vi "SI657_From_trubine.vi"(0 "From Turbine SI656":T1, 2 "From Turbine SI657":T2, 5 "error in (no error)":errorcluster, 8 "SI657.lvclass":refnum<class "SI657.lvclass">, 10 "SI656.lvclass":refnum<class "SI656.lvclass">) -> (9 "SI657.lvclass out":refnum<class "SI657.lvclass">, 11 "SI656 out":refnum<class "SI656.lvclass">, 14 "PG SP-Grad":dbl, 15 "PG SP lift-up":dbl, 16 "PG eff SP":dbl, 17 "Switch Ps-Ps_d":dbl, 18 "PG target SP":dbl, 19 "error out":errorcluster)   [LabVIEW 2022 SP3, in "SI657.lvclass"]
uses:
  SI657.lvclass
  SI657.lvclass/SI657.ctl
  SI656/SI656.lvclass
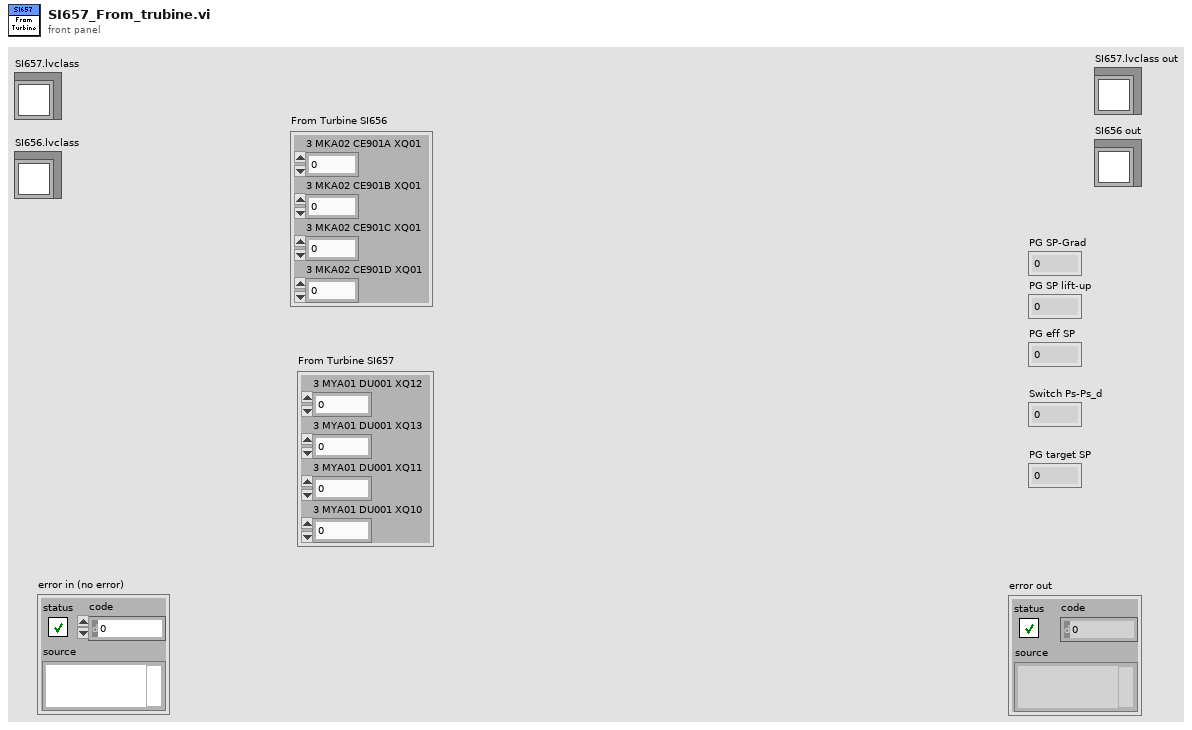
[diagram p1: front panel]
types:
  T1 = cluster{"3 MKA02 CE901A XQ01":dbl, "3 MKA02 CE901B XQ01":dbl, "3 MKA02 CE901C XQ01":dbl, "3 MKA02 CE901D XQ01":dbl}
  T2 = cluster{"3 MYA01 DU001 XQ12":dbl, "3 MYA01 DU001 XQ13":dbl, "3 MYA01 DU001 XQ11":dbl, "3 MYA01 DU001 XQ10":dbl}
  T3 = cluster{"UL":dbl, "LL":dbl, "OutLimMax":dbl, "OutLimMin":dbl}
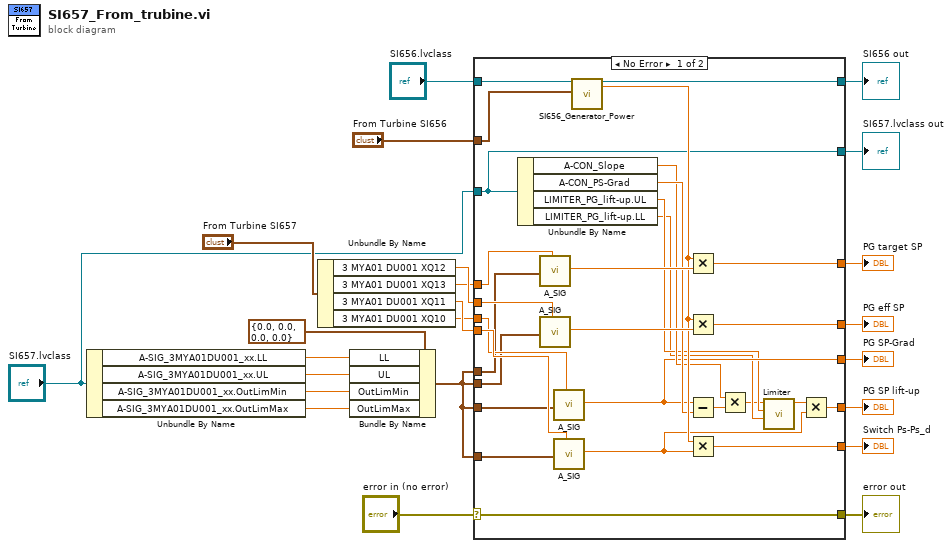
[diagram p0: block diagram]
diagram:
  n1 = Unbundle By Name("SI657.lvclass") -> ("A-SIG_3MYA01DU001_xx.LL"=w5:dbl, "A-SIG_3MYA01DU001_xx.UL"=w4:dbl, "A-SIG_3MYA01DU001_xx.OutLimMin"=w3:dbl, "A-SIG_3MYA01DU001_xx.OutLimMax"=w2:dbl)
  n2 = Unbundle By Name("From Turbine SI657") -> ("3 MYA01 DU001 XQ12"=w12:dbl, "3 MYA01 DU001 XQ13"=w11:dbl, "3 MYA01 DU001 XQ11"=w10:dbl, "3 MYA01 DU001 XQ10"=w9:dbl)
  n3 = Bundle By Name(cluster=T3 {"UL"=0.0, "LL"=0.0, "OutLimMax"=0.0, "OutLimMin"=0.0} ("Set Params"), "LL"=w5, "UL"=w4, "OutLimMin"=w3, "OutLimMax"=w2) -> (w1:T3)
  n4 = case shown="No Error" "error in (no error)" {
    selector: "error in (no error)" -> [w52 w53]
    tunnel: [w52 w53] -> w22
    tunnel: w12 -> [w51 _]
    tunnel: w11 -> [w50 _]
    tunnel: w10 -> [w49 _]
    tunnel: w9 -> [w48 _]
    tunnel: "SI657.lvclass" -> [w39 _]
    tunnel: [w39 _] -> w21
    tunnel: "SI656.lvclass" -> [w47 _]
    tunnel: [w46 _] -> w19
    tunnel: [w44 _] -> w18
    tunnel: [w42 _] -> w17
    tunnel: [w40 _] -> w16
    tunnel: [w35 _] -> w15
    tunnel: [w29 _] -> w14
    tunnel: "From Turbine SI656" -> [w28 _]
    tunnel: w1 -> [w27 _]
    tunnel: w1 -> [w26 _]
    tunnel: w1 -> [w25 _]
    tunnel: w1 -> [w24 _]
    frame No Error {
      n5 = Unbundle By Name(w39) -> ("A-CON_Slope"=w36:dbl, "A-CON_PS-Grad"=w38:dbl, "LIMITER_PG_lift-up.UL"=w34:dbl, "LIMITER_PG_lift-up.LL"=w33:dbl)
      n6 = call "A_SIG.vi"("Set Params"=w24, "Input"=w50) -> ("A_SIG_out"=w43:dbl)  [unwired: 16 in, 1 out]
      n7 = call "A_SIG.vi"("Set Params"=w25, "Input"=w51) -> ("A_SIG_out"=w45:dbl)  [unwired: 16 in, 1 out]
      n8 = call "A_SIG.vi"("Set Params"=w27, "Input"=w48) -> ("A_SIG_out"=w35:dbl)  [unwired: 16 in, 1 out]
      n9 = call "A_SIG.vi"("Set Params"=w26, "Input"=w49) -> ("A_SIG_out"=w31:dbl)  [unwired: 16 in, 1 out]
      n10 = call "SI656_Generator_Power.vi"("SI656 in"=w47, "From Turbine"=w28) -> ("SI656 out"=w46:refnum<class "SI656.lvclass">, "PG Factor"=w41:dbl)  [unwired: 14 in, 2 out]
      n11 = Multiply(x=w41, y=w43) -> (x*y=w42:dbl)
      n12 = Multiply(x=w41, y=w45) -> (x*y=w44:dbl)
      n13 = Subtract(x=w35, y=w38) -> (x-y=w37:dbl)
      n14 = Multiply(x=w41, y=w31) -> (x*y=w40:dbl)
      n15 = Multiply(x=w36, y=w37) -> (x*y=w32:dbl)
      n16 = call "Limiter.vi"("LIMITER_PG_lift-up.LL"=w33, "LIMITER_PG_lift-up.UL in"=w34, "input"=w32) -> ("LIMITER_PG_lift-up.UL out"=w30:dbl)  [unwired: 7 in, 1 out]
      n17 = Multiply(x=w30, y=w31) -> (x*y=w29:dbl)
    }
    frame Error {
    }
  }
  "error out" <- w22
  "SI657.lvclass out" <- w21
  "SI656 out" <- w19
  "PG eff SP" <- w18
  "PG target SP" <- w17
  "Switch Ps-Ps_d" <- w16
  "PG SP-Grad" <- w15
  "PG SP lift-up" <- w14
